vi "Write DAQ Type.vi"(8 "error in (no error)":errorcluster, 10 "Type":enum16{"Hardware", "Simulation"}(ring), 11 "BK-Precision in":refnum<class "BK-Precision.lvclass">) -> (0 "error out":errorcluster, 3 "BK-Precision out":refnum<class "BK-Precision.lvclass">)   [LabVIEW 2016, in "DC PWS.lvlib" / "BK-Precision.lvclass"]
uses:
  BK-Precision.lvclass
  BK-Precision.lvclass/BK-Precision.ctl
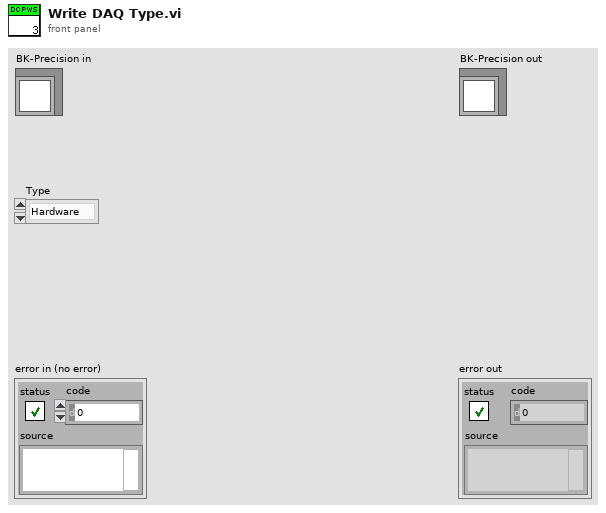
[diagram p1: front panel]
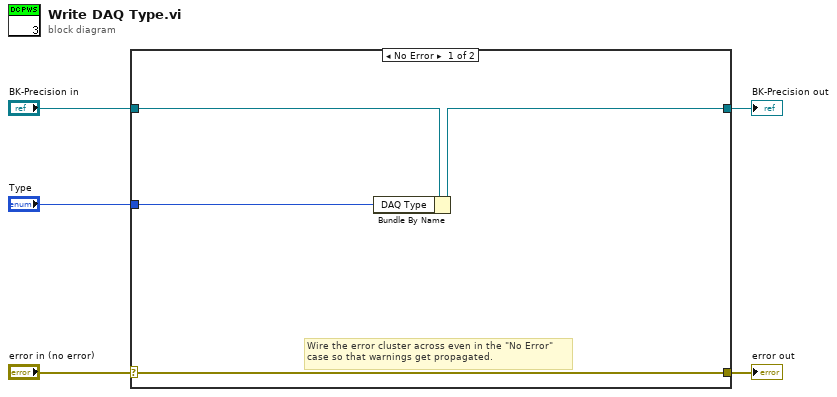
[diagram p0: block diagram]
diagram:
  n1 = case shown="No Error" "error in (no error)" {
    selector: "error in (no error)" -> [w8 w11]
    tunnel: [w8 w11] -> w4
    tunnel: [w7 w10] -> w2
    tunnel: "BK-Precision in" -> [w9 w10]
    tunnel: "Type" -> [w6 _]
    frame No Error {
      # "Wire the error cluster across even in the \"No Error\"\ncase so that warnings get propagated."
      n2 = Bundle By Name(cluster=w9, "DAQ Type"=w6) -> (w7:refnum<class "BK-Precision.lvclass">)
    }
    frame Error {
    }
  }
  "error out" <- w4
  "BK-Precision out" <- w2
